vi "Add to Sector Accumulation.vi"(9 "[Accumulated Sectors] In":T1[](array[typedef]), 10 "Pixel Intensity":u8, 11 "Sector ID":u8) -> (3 "[Accumulated Sectors] Out":T1[](array[typedef]))   [LabVIEW 2013]
uses:
  FPGA/Sector/Accumulate/Accumulated Sector Cluster.ctl
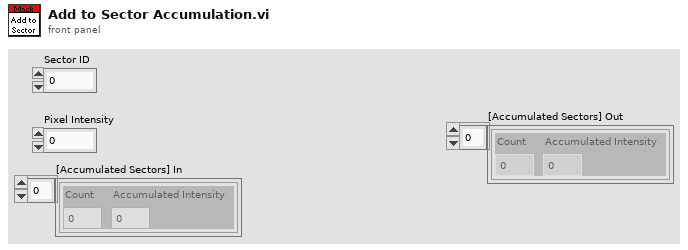
[diagram p1: front panel]
types:
  T1 = typedef "Accumulated Sector Cluster.ctl" = cluster{"Accumulated Intensity":u32, "Count":u16}
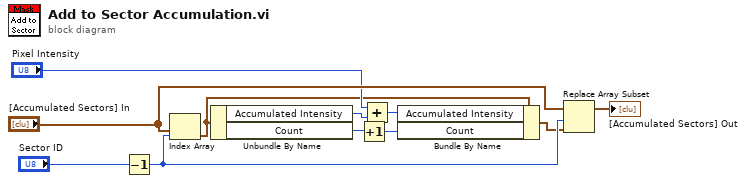
[diagram p0: block diagram]
diagram:
  n1 = Decrement(x="Sector ID") -> (x-1=w7:u8)
  n2 = Index Array(array="[Accumulated Sectors] In", index=w7) -> (element=w2:T1)
  n3 = Unbundle By Name(w2) -> ("Accumulated Intensity"=w9:u32, "Count"=w11:u16)
  n4 = Increment(x=w11) -> (x+1=w10:u16)
  n5 = Add(x="Pixel Intensity", y=w9) -> (x+y=w8:u32)
  n6 = Bundle By Name(cluster=w2, "Accumulated Intensity"=w8, "Count"=w10) -> (w1:T1)
  n7 = Replace Array Subset(array="[Accumulated Sectors] In", new element=w1, index=w7) -> (→"[Accumulated Sectors] Out":T1[])
